vi "Build Major Frame Schedule.vi"(7 "Virtual Memory Unit in":refnum<class "Virtual Memory Unit.lvclass">, 8 "error in (no error)":errorcluster, 10 "Starting Address":u16 format="%04x", 11 "Major Frame in":refnum<class "Major Frame.lvclass">) -> (0 "error out":errorcluster, 2 "Next Available Address":u16 format="%04x", 3 "Major Frame out":refnum<class "Major Frame.lvclass">, 4 "Final Data Address":u16 format="%04x", 5 "Virtual Memory Unit out":refnum<class "Virtual Memory Unit.lvclass">)   [LabVIEW 2020, in "BCI-1553 API.lvlib" / "Major Frame.lvclass"]
doc: "Assesses the estimate size of the Major Frame block. Pops an ID off of the Major Frame Schedule and identifies it as a Minor Frame or a Message. Depending on this analysis, a Message or Minor Frame will be added in sequence to this Major Frame."
uses:
  Major Frame.lvclass
  Dependencies/Virtual Memory Unit/Virtual Memory Unit.lvclass
  Major Frame.lvclass/Major Frame.ctl
  TypeDefs/Minor Frame Pointers.ctl
  TypeDefs/Message Pointers.ctl
  Minor Frame/Minor Frame.lvclass
  BCI-1553 API.lvlib
  Message/Message.lvclass
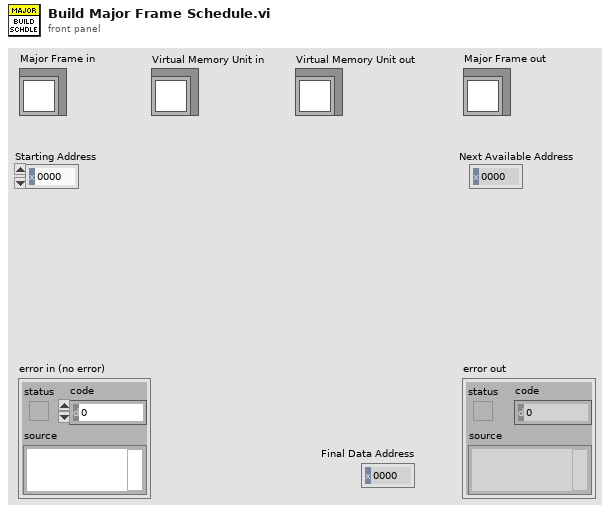
[diagram p1: front panel]
types:
  T1 = typedef "BCI-1553 API.lvlib/Message Pointers.ctl" = cluster{"SubRoutine Address":u16, "HP Async Address":u16}
  T2 = typedef "BCI-1553 API.lvlib/Minor Frame Pointers.ctl" = cluster{"SubRoutine Address":u16, "Next Frame Address":u16, "HP Async Address":u16}
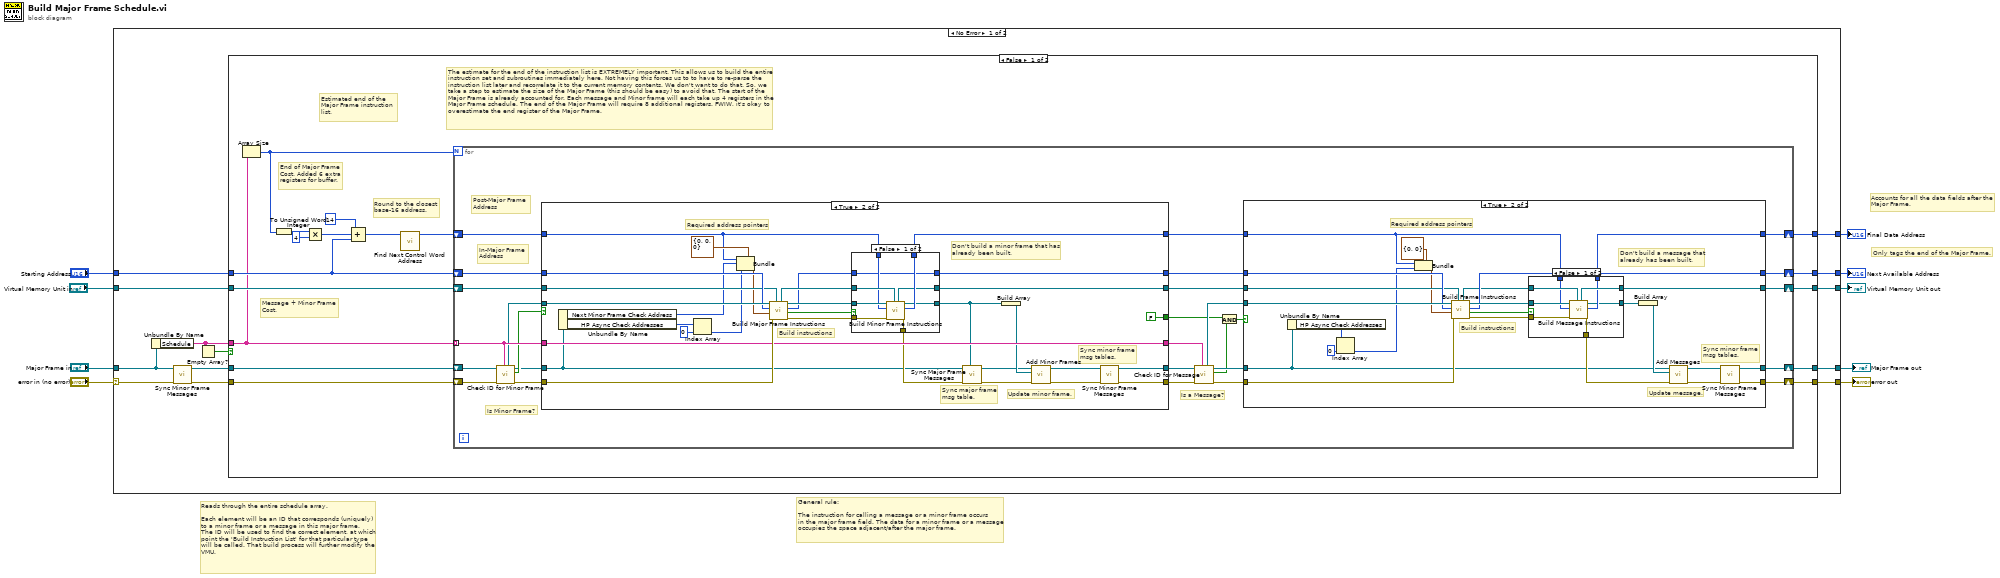
[diagram p0: block diagram]
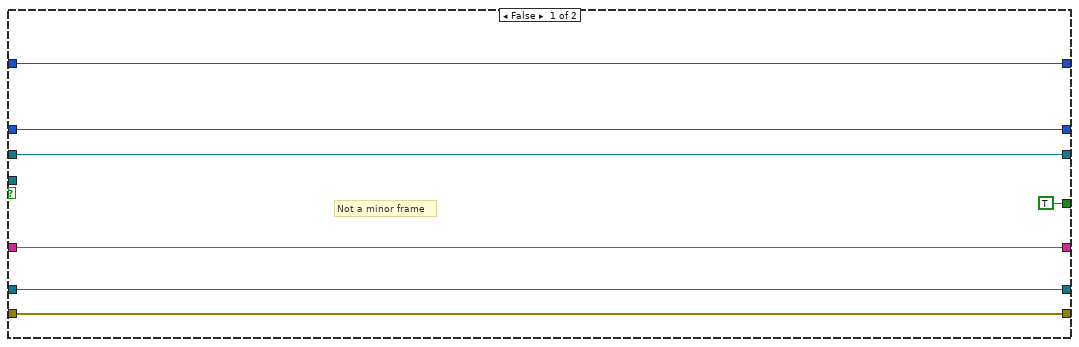
[diagram p4: hidden frame]
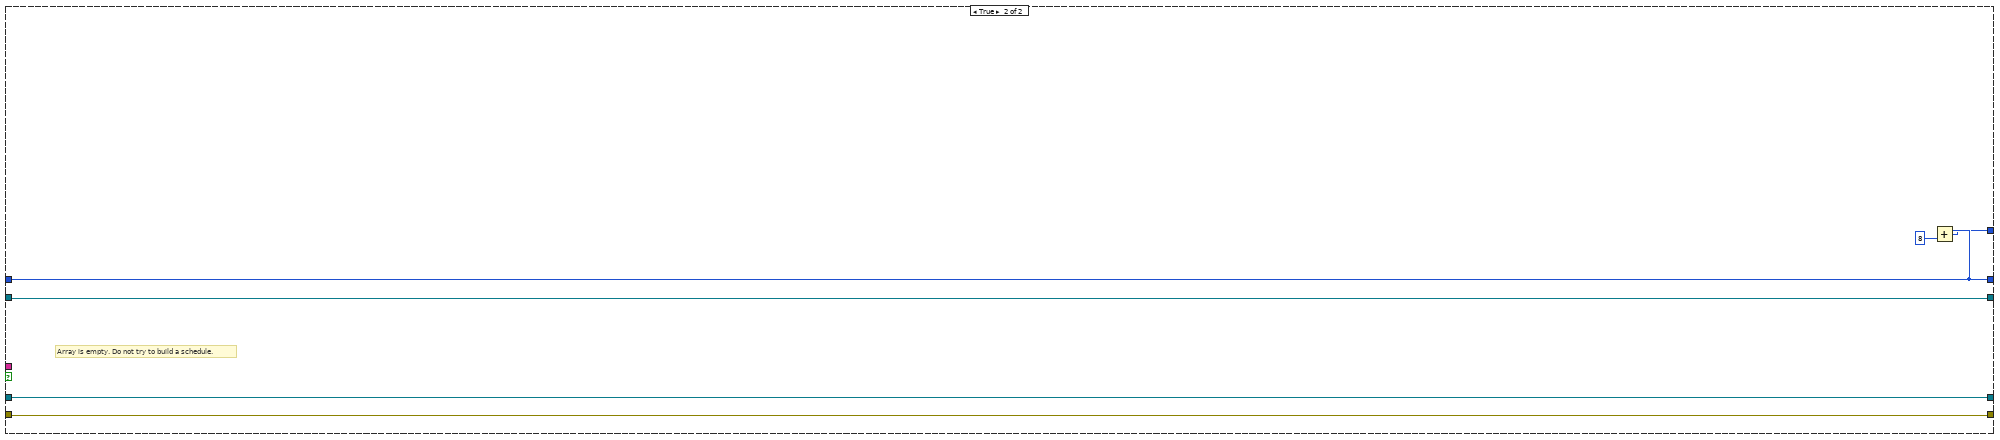
[diagram p6: hidden frame]
diagram:
  # "General rule:\n\nThe instruction for calling a message or a minor frame occurs\nin the major frame field. The data for a minor frame or a message \noccupies the space adjacent/after the major frame."
  # "Only tags the end of the Major Frame."
  # "Accounts for all the data fields after the\nMajor Frame."
  # "Reads through the entire schedule array.\n\nEach element will be an ID that corresponds (uniquely)\nto a minor frame or a message in this major frame.\nThe ID will be used to find the correct element, at which\npoint the 'Build Instruction List' for that particular type\nwill be called. That build process will further modify the\nVMU."
  n1 = case shown="No Error" "error in (no error)" {
    selector: "error in (no error)" -> [w14 w170]
    tunnel: [w22 w170] -> w8
    tunnel: [w21 w169] -> w6
    tunnel: "Major Frame in" -> [w16 w169]
    tunnel: "Virtual Memory Unit in" -> [w20 w168]
    tunnel: [w18 w168] -> w4
    tunnel: "Starting Address" -> [w17 w167]
    tunnel: [w19 w167] -> w2
    tunnel: [w10 _] -> w1
    frame No Error {
      n2 = Unbundle By Name(w16) -> ("Schedule"=w12:string[])
      n3 = call "Sync Minor Frame Messages.vi"("error in (no error)"=w14, "Major Frame in"=w16) -> ("error out"=w13:errorcluster, "Major Frame out"=w15:refnum<class "Major Frame.lvclass">)  [unwired: 8 in]
      n4 = Empty Array?(array=w12) -> (empty?=w11:bool)
      n5 = case shown="False" w11 {
        tunnel: [w39 w164] -> w22
        tunnel: [w38 w165] -> w21
        tunnel: w20 -> [w37 w166]
        tunnel: [w36 w163] -> w19
        tunnel: [w35 w166] -> w18
        tunnel: w17 -> [w31 w163]
        tunnel: w15 -> [w27 w165]
        tunnel: w13 -> [w26 w164]
        tunnel: w12 -> [w24 _]
        tunnel: [w25 w162] -> w10
        frame False {
          # "Round to the closest\nbase-16 address."
          # "End of Major Frame\nCost. Added 6 extra\nregisters for buffer."
          # "Message + Minor Frame\nCost."
          # "The estimate for the end of the instruction list is EXTREMELY important. This allows us to build the entire\ninstruction set and subroutines immediately here. Not having this forces us to to have to re-parse the\ninstruction list later and recorrelate it to the current memory contents. We don't want to do that. So, we\ntake a step to estimate the size of the Major Frame (this should be easy) to avoid that. The start of the \nMajor Frame is already accounted for. Each message and Minor frame will each take up 4 registers in the\nMajor Frame schedule. The end of the Major Frame will require 8 additional registers. FWIW, it's okay to\noverestimate the end register of the Major Frame."
          # "Estimated end of the\nMajor Frame instruction\nlist."
          n6 = Array Size(array=w24) -> (size(s)=w23:i32)
          n7 = To Unsigned Word Integer(number=w23) -> (unsigned 16bit integer=w34:u16)
          n8 = Multiply(x=w34, y=u16 4) -> (x*y=w32:u16)
          n9 = Compound Arithmetic op=ADD(u16 14 ("value"), w32, w31) -> (w29:u16)
          n10 = call "Find Next Control Word Address.vi"("Starting Address"=w29) -> ("0xHHHX Address"=w28:u16)  [unwired: 10 in]
          n11 = for {
            N: w23 -> [_]
            shift-right: [w66] -> w39
            shift-left: w26 -> [w56]
            shift-right: [w65] -> w38
            shift-left: w27 -> [w58]
            shift-right: [w62] -> w35
            shift-left: w37 -> [w61]
            shift-right: [w64] -> w36
            shift-left: w31 -> [w63]
            tunnel: w24 -> [w57] mode=indexing
            shift-right: [w60] -> w25
            shift-left: w28 -> [w59]
            # "Is a Message?"
            # "Is Minor Frame?"
            # "In-Major Frame\nAddress"
            # "Post-Major Frame\nAddress"
            n12 = call "Check ID for Minor Frame.vi"("ID"=w57, "error in (no error)"=w56, "Major Frame in"=w58) -> ("error out"=w46:errorcluster, "Minor Frame Found?"=w55:bool, "Major Frame out"=w47:refnum<class "Major Frame.lvclass">, "Minor Frame"=w54:refnum<class "Minor Frame.lvclass">)  [unwired: 5 in]
            n13 = case shown="True" w55 {
              tunnel: w54 -> [_ w145]
              tunnel: w61 -> [w114 w143]
              tunnel: w63 -> [w113 w144]
              tunnel: w59 -> [w112 w133]
              tunnel: w46 -> [w115 w146]
              tunnel: [w115 w125] -> w52
              tunnel: [w114 w137] -> w50
              tunnel: [w113 w117] -> w49
              tunnel: [w112 w139] -> w48
              tunnel: w47 -> [w110 w122]
              tunnel: w57 -> [w111 w142]
              tunnel: [w111 w142] -> w43
              tunnel: [w110 w127] -> w44
              tunnel: [TRUE FALSE] -> w42
              frame False {
                # "Not a minor frame"
              }
              frame True {
                # "Don't build a minor frame that has\nalready been built."
                # "Sync major frame\nmsg table."
                # "Sync minor frame\nmsg tables."
                # "Required address pointers"
                # "Update minor frame."
                # "Build instructions"
                n14 = Unbundle By Name(w122) -> ("Next Minor Frame Check Address"=w132:u16, "HP Async Check Addresses"=w130:u16[])
                n15 = Index Array(array=w130, index=0) -> (element=w129:u16)
                n16 = Bundle(cluster=T2 {"SubRoutine Address"=0, "Next Frame Address"=0, "HP Async Address"=0} ("Minor Frame Pointers"), "SubRoutine Address"=w133, "Next Frame Address"=w132, "HP Async Address"=w129) -> (w134:T2)
                n17 = call-dynamic "Build Major Frame Instructions.vi"("Virtual Memory Unit in"=w143, "error in (no error)"=w146, "Minor Frame Pointers"=w134, "Starting Address"=w144, "Minor Frame in"=w145) -> ("error out"=w140:errorcluster, "Already Config'd"=w119:bool, "Next Available Address"=w118:u16, "Minor Frame out"=w141:refnum<class "Minor Frame.lvclass">, "Virtual Memory Unit out"=w138:refnum<class "Virtual Memory Unit.lvclass">)  [unwired: 2 in]
                n18 = case shown="False" w119 {
                  tunnel: w141 -> [w155 w157]
                  tunnel: w140 -> [w154 w156]
                  tunnel: [w153 w160] -> w139
                  tunnel: w138 -> [w152 w159]
                  tunnel: [w151 w159] -> w137
                  tunnel: w133 -> [w150 w160]
                  tunnel: [w149 w156] -> w124
                  tunnel: [w148 w157] -> w120
                  tunnel: w118 -> [w147 w158]
                  tunnel: [w147 w158] -> w117
                  frame False {
                    n19 = call-dynamic "Build Minor Frame Instructions.vi"("Virtual Memory Unit in"=w152, "error in (no error)"=w154, "Starting Address"=w150, "Minor Frame in"=w155) -> ("error out"=w149:errorcluster, "Next Available Address"=w153:u16, "Minor Frame out"=w148:refnum<class "Minor Frame.lvclass">, "Virtual Memory Unit out"=w151:refnum<class "Virtual Memory Unit.lvclass">)  [unwired: 4 in]
                  }
                  frame True {
                  }
                }
                n20 = call "Sync Major Frame Messages.vi"("Minor Frame"=w120, "error in (no error)"=w124, "Major Frame in"=w122) -> ("error out"=w123:errorcluster, "Major Frame out"=w121:refnum<class "Major Frame.lvclass">)  [unwired: 7 in]
                n21 = Build Array(w120) -> (w136:refnum<class "Minor Frame.lvclass">[])
                n22 = call-dynamic "Add Minor Frames.vi"("error in (no error)"=w123, "Minor Frames"=w136, "Major Frame in"=w121) -> ("error out"=w126:errorcluster, "Major Frame out"=w128:refnum<class "Major Frame.lvclass">)  [unwired: 7 in]
                n23 = call "Sync Minor Frame Messages.vi"("error in (no error)"=w126, "Major Frame in"=w128) -> ("error out"=w125:errorcluster, "Major Frame out"=w127:refnum<class "Major Frame.lvclass">)  [unwired: 8 in]
              }
            }
            n24 = call "Check ID for Message.vi"("ID"=w43, "error in (no error)"=w52, "Major Frame in"=w44) -> ("error out"=w51:errorcluster, "Msg Found?"=w41:bool, "Major Frame out"=w45:refnum<class "Major Frame.lvclass">, "Message"=w53:refnum<class "Message.lvclass">)  [unwired: 5 in]
            n25 = And(x=w42, y=w41) -> (x .and. y?=w40:bool)
            n26 = case shown="True" w40 {
              tunnel: w53 -> [_ w96]
              tunnel: w51 -> [w68 w93]
              tunnel: [w68 w72] -> w66
              tunnel: w50 -> [w69 w90]
              tunnel: [w69 w88] -> w62
              tunnel: [w70 w91] -> w64
              tunnel: w49 -> [w70 w92]
              tunnel: [w71 w87] -> w60
              tunnel: w48 -> [w71 w82]
              tunnel: w45 -> [w67 w80]
              tunnel: [w67 w74] -> w65
              frame False {
                # "Not a message"
              }
              frame True {
                # "Don't build a message that\nalready has been built."
                # "Sync minor frame\nmsg tables."
                # "Required address pointers"
                # "Update message."
                # "Build instructions"
                n27 = Unbundle By Name(w80) -> ("HP Async Check Addresses"=w79:u16[])
                n28 = Index Array(array=w79, index=0) -> (element=w77:u16)
                n29 = Bundle(cluster=T1 {"SubRoutine Address"=0, "HP Async Address"=0} ("Message Pointers"), "SubRoutine Address"=w82, "HP Async Address"=w77) -> (w81:T1)
                n30 = call "Build Frame Instructions.vi"("Virtual Memory Unit in"=w90, "error in (no error)"=w93, "Message Pointers"=w81, "Starting Address"=w92, "Message in"=w96) -> ("error out"=w94:errorcluster, "Msg Already Configured"=w76:bool, "Next Available Address"=w91:u16, "Message out"=w95:refnum<class "Message.lvclass">, "Virtual Memory Unit out"=w89:refnum<class "Virtual Memory Unit.lvclass">)  [unwired: 2 in]
                n31 = case shown="False" w76 {
                  tunnel: w95 -> [w104 w106]
                  tunnel: w94 -> [w103 w105]
                  tunnel: w89 -> [w102 w107]
                  tunnel: [w101 w107] -> w88
                  tunnel: [w100 w108] -> w87
                  tunnel: [w99 w106] -> w86
                  tunnel: [w98 w105] -> w84
                  tunnel: w82 -> [w97 w108]
                  frame False {
                    n32 = call "Build Message Instructions.vi"("Virtual Memory Unit in"=w102, "error in (no error)"=w103, "Starting Address"=w97, "Message in"=w104) -> ("error out"=w98:errorcluster, "Next Available Address"=w100:u16, "Message out"=w99:refnum<class "Message.lvclass">, "Virtual Memory Unit out"=w101:refnum<class "Virtual Memory Unit.lvclass">)  [unwired: 4 in]
                  }
                  frame True {
                  }
                }
                n33 = Build Array(w86) -> (w85:refnum<class "Message.lvclass">[])
                n34 = call-dynamic "Add Messages.vi"("error in (no error)"=w84, "Messages"=w85, "Major Frame in"=w80) -> ("error out"=w73:errorcluster, "Major Frame out"=w75:refnum<class "Major Frame.lvclass">)  [unwired: 7 in]
                n35 = call "Sync Minor Frame Messages.vi"("error in (no error)"=w73, "Major Frame in"=w75) -> ("error out"=w72:errorcluster, "Major Frame out"=w74:refnum<class "Major Frame.lvclass">)  [unwired: 8 in]
              }
            }
          }
        }
        frame True {
          # "Array is empty. Do not try to build a schedule."
          n36 = Add(x=w163, y=u16 8) -> (x+y=w162:u16)
        }
      }
    }
    frame Error {
    }
  }
  "error out" <- w8
  "Major Frame out" <- w6
  "Virtual Memory Unit out" <- w4
  "Next Available Address" <- w2
  "Final Data Address" <- w1
